vi "Measurement UI.vi"() -> ()   [LabVIEW 2021, in "Efficiency And Load Regulation with Pin Map UI.lvlib"]
uses:
  Efficiency And Load Regulation with Pin Map UI.lvlib
  <instrlib>/niScope/Controls/niScope vertical coupling.ctl
  <instrlib>/niDMM/nidmm.llb/niDMM Resolution in Digits.ctl
  subVIs/UI Controls.ctl
  common/UI/controls/UI Scope Parameters.ctl
  common/UI/controls/UI DMM Parameters.ctl
  d93153ab-98af-4bc3-81b9-2719e6b72da3.vi
  common/PMIC Common.lvlib
panel:
  in  "MeasGraphs":T1(tab)
  out "EfficiencyGraph 2":T2(graph)
  out "EfficiencyGraph":T2(graph)
  out "LoadRegulationGraph(V/A)":T2(graph)
  out "LoadRegulationGraph(%)":T2(graph)
  in  "dmm function array":u32[](array[ring]) items=["DC Volts", "AC Volts", "DC Current", "AC Current", "2-wire Resistance", "4-wire Resistance", "Diode", "Frequency", "Period", "AC Volts DC Coupled", "Capacitance", "Inductance", "Temperature"]
  in  "dmm range array":dbl[](array[numeric])
  in  "dmm resolution in digits array":T3[](array[typedef]) items=["3 1/2"=3.5, "4 1/2"=4.5, "5 1/2"=5.5, "6 1/2"=6.5, "7 1/2"=7.5]
  in  "dmm pin names":string[](array[string])
  in  "Source voltage array size":i32[](array[numeric])
  in  "Source voltage concatenated array":dbl[](array[numeric]) caption="VOLTAGE ARRAY"
  out "waveform pins":string[](array[string])
  in  "enforce realtime":bool[](array[boolean])
  in  "reference position":dbl[](array[numeric]) caption="MIN SAMPLE RATE"
  in  "channel enabled":bool[](array[boolean])
  out "waveform length array":i32[](array[numeric])
  out "waveform dt array":dbl[](array[numeric])
  out "Maximum load regulation":dbl[](array[numeric])
  out "Minimum load regulation":dbl[](array[numeric])
  out "Maximum load voltage":dbl[](array[numeric])
  out "Minimum load voltage":dbl[](array[numeric])
  out "Maximum efficiency":dbl[](array[numeric])
  out "Minimum efficiency":dbl[](array[numeric])
  out "Source sweep points":i32
  out "Load voltage deviation":dbl[](array[numeric])
  out "Load voltages":dbl[](array[numeric])
  out "Voltage values":dbl[](array[numeric])
  out "Load sweep points":i32
  out "Efficiency":dbl[](array[numeric])
  out "Load currents":dbl[](array[numeric])
  out "concatenated waveform Y":dbl[](array[numeric])
  out "waveform t0 array":dbl[](array[numeric])
  out "waveform sites":i32[](array[numeric])
  in  "vertical range":dbl[](array[numeric]) caption="VERTICAL RANGE"
  in  "vertical offset":dbl[](array[numeric]) caption="VERTICAL OFFSET"
  in  "probe attenuation":dbl[](array[numeric]) caption="PROBE ATTENUATION"
  in  "vertical coupling":T4[](array[typedef]) caption="VERTICAL COUPLING" items=["AC", "DC", "Ground"]
  in  "input impedance":u32[](array[ring]) caption="INPUT IMPEDANCE" items=["1 mega ohm"=0, "50 ohms"=2]
  in  "max input frequency":dbl[](array[numeric]) caption="MAX INPUT FREQUENCY"
  in  "min sample rate":dbl[](array[numeric]) caption="MIN SAMPLE RATE"
  in  "min record length":i32[](array[numeric]) caption="MIN RECORD LENGTH"
  in  "Pin Names for Scope":string[](array[string]) caption="PIN NAMES"
  out "MeasTable":string[][](table)
  in  "Source pin name index for efficiency":i32 caption="PIN INDEX USED IN EFFICIENCY CALCULATION"
  in  "Source stop voltage array":dbl[](array[numeric])=[20.0] caption="STOP VOLTAGE" format="%#_6pV"
  in  "Source start voltage array":dbl[](array[numeric])=[6.0] caption="START VOLTAGE" format="%#_6pV"
  in  "Source maximum power array":dbl[](array[numeric])=[300.0] caption="SOURCE MAXIMUM POWER" format="%#_6pW"
  in  "Source current limit array":dbl[](array[numeric])=[25.0] caption="SOURCE CURRENT LIMIT" format="%#_6pA"
  in  "Source sense array":i32[](array[ring])=[1009] caption="SOURCE SENSE" items=["Local"=1008, "Remote"=1009]
  in  "Source pin name array":string[](array[string]) caption="SOURCE PIN NAMES"
  in  "Open DMM Dialog":bool
  in  "DMM configuration":string="DMM configuration"
  in  "Open Scope Dialog":bool
  in  "Load pin name":string caption="LOAD PIN NAME"
  in  "Use Load current array":bool caption="USE ARRAY?"
  in  "Load current array":dbl[](array[numeric]) caption="CURRENT ARRAY"
  in  "Source voltage array":dbl[][](array[numeric]) caption="VOLTAGE ARRAY"
  in  "Use Source voltage array":bool caption="USE ARRAY?"
  in  "Scope configuration":string="Scope configuration"
  in  "Load sense":i32(ring)=1009 caption="SENSE" items=["Local"=1008, "Remote"=1009]
  out "Status":string
  in  "Load sweep type":string(combo)="Logarithmic" caption="SWEEP TYPE"
  in  "DUT setup time":dbl=1.0 caption="DUT SETUP TIME" format="%#_6ps"
  in  "Source voltage sweep points":i32=4 caption="NO. OF POINTS"
  in  "Aperture time":dbl=0.005 caption="APERTURE TIME" format="%#_6ps"
  in  "Source delay":dbl=0.005 caption="SOURCE DELAY" format="%#_6ps"
  in  "Load current sweep points/points per decade":i32=10 caption="PTS/PTS PER DECADE"
  in  "Load stop current":dbl=24.0 caption="STOP CURRENT" format="%#_6pA"
  in  "Load start current":dbl=0.1 caption="START CURRENT" format="%#_6pA"
  in  "Load voltage limit range":dbl=6.0 caption="VOLTAGE LIMIT RANGE" format="%#_6pV"
  in  "Load configuration":string="Load configuration"
  in  "Source configuration":string="Source configuration"
  in  "Measurement settings":string="Measurement settings"
  in  "Nominal output voltage":dbl=3.3 caption="NOMINAL OUTPUT VOLTAGE" format="%#_6pV"
  in  "Mode of operation":T5(ring)=enum."Perform measurement" caption="MODE OF OPERATION"
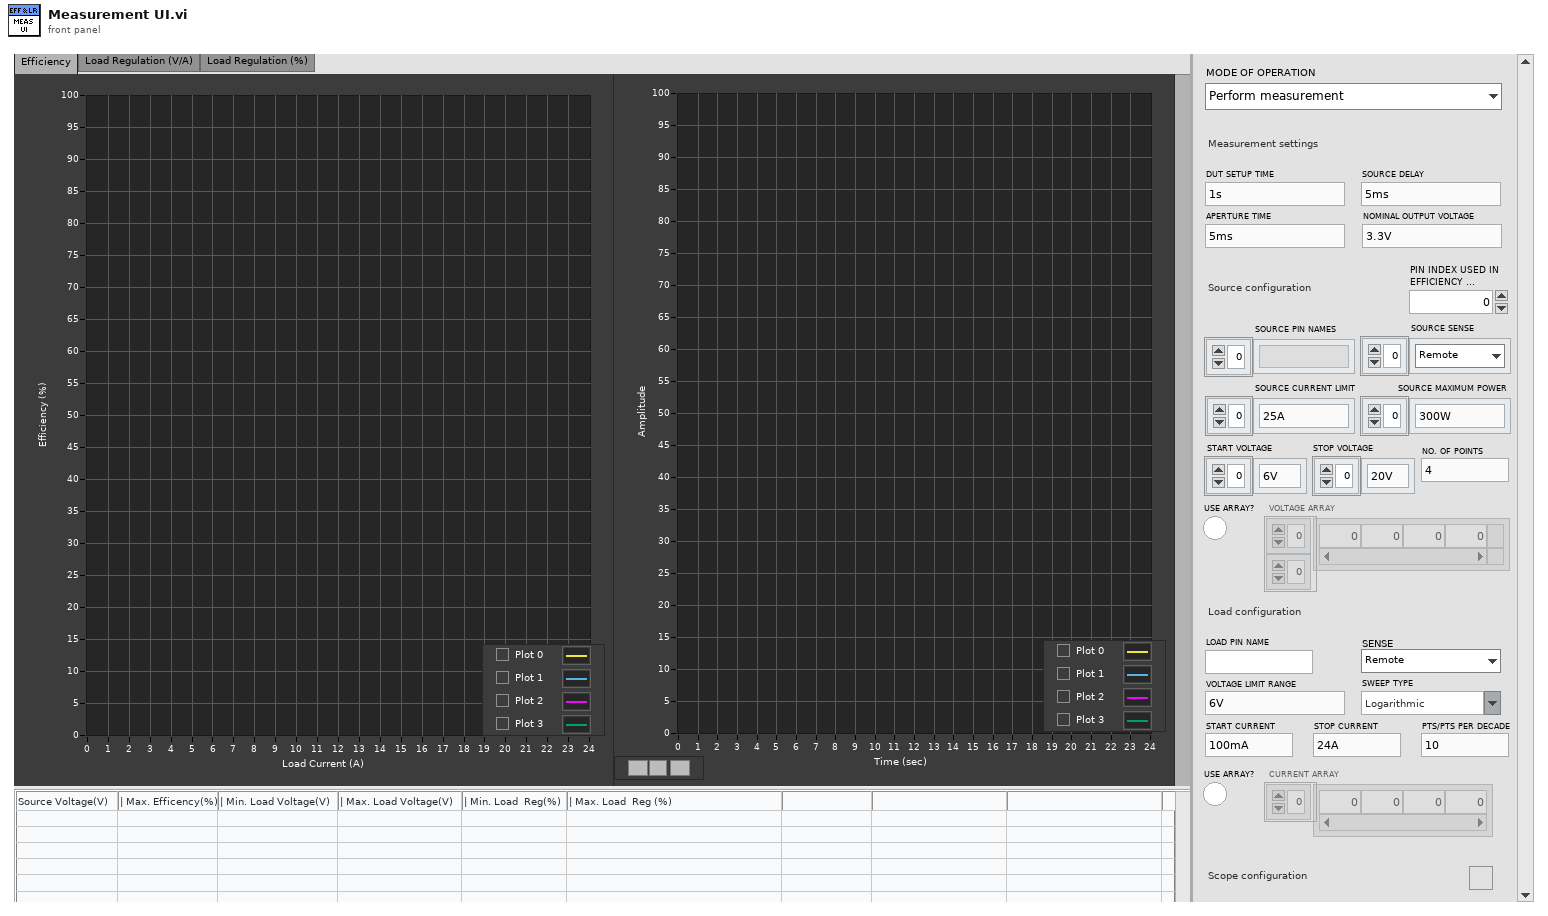
[diagram p1: front panel]
types:
  T1 = enum32{"Efficiency", "Load Regulation (V/A)", "Load Regulation (%)", "Hidden Controls"}
  T2 = cluster{"Load currents":dbl[], "Efficiency":dbl[]}[]
  T3 = typedef "niDMM Resolution in Digits.ctl" = dbl
  T4 = typedef "niScope vertical coupling.ctl" = i32
  T5 = enum32{"Power on the DUT", "Perform measurement", "Power off the DUT"}
  T6 = typedef "PMIC Common.lvlib/UI Scope Parameters.ctl" = cluster{"Pin name":string, "Vertical range":dbl, "Vertical offset":dbl, "Probe attenuation":dbl, "Vertical coupling":i32, "Channel enabled":bool, "Input impedance":u32, "Max input frequency":dbl, "Min sample rate":dbl, "Reference position":dbl, "Min record length":i32, "Enforce realtime":bool}
  T7 = typedef "PMIC Common.lvlib/UI DMM Parameters.ctl" = cluster{"Pin name":string, "Function":u32, "Resolution in Digits":dbl, "Range":dbl}
  T8 = enum8{"Enabled", "Disabled", "Disabled and Grayed Out"}
  T9 = typedef "Efficiency And Load Regulation with Pin Map UI.lvlib/UI Controls.ctl" = enum16{"", "EfficiencyGraph", "LoadRegulationGraph(V/A)", "LoadRegulationGraph(%)", "ScopeGraph", "DUT setup time", "Source delay", "Aperture time", "Nominal output voltage", "Source pin name", "Source current limit", "Source maximum power", "Source start voltage", "Source stop voltage", "Source voltage sweep points", "Load pin name", "Load voltage limit range", "Load sweep type", "Load start current", "Load stop current", "Load current sweep points/points per decade", "Use Load current array", "Load current array", "Use Source voltage array", "Source voltage array", "Pin Names for Scope", "vertical range", "vertical offset", "probe attenuation", "vertical coupling", "channel enabled", "input impedance", "max input frequency", "min sample rate", "reference position", "min record length", "enforce realtime", "Measurement settings", "Source configuration", "Load configuration", "Source sense", "Load sense", "Scope configuration", "Open Scope Dialog", "DMM configuration", "Open DMM Dialog", "Source pin name index for efficiency"}
  T10 = cluster{"Load currents":dbl[], "Efficiency":dbl[]}
  T11 = cluster{"Load currents":dbl[], "Load voltages":dbl[]}
  T12 = cluster{"Load currents":dbl[], "Load voltage deviation":dbl[]}
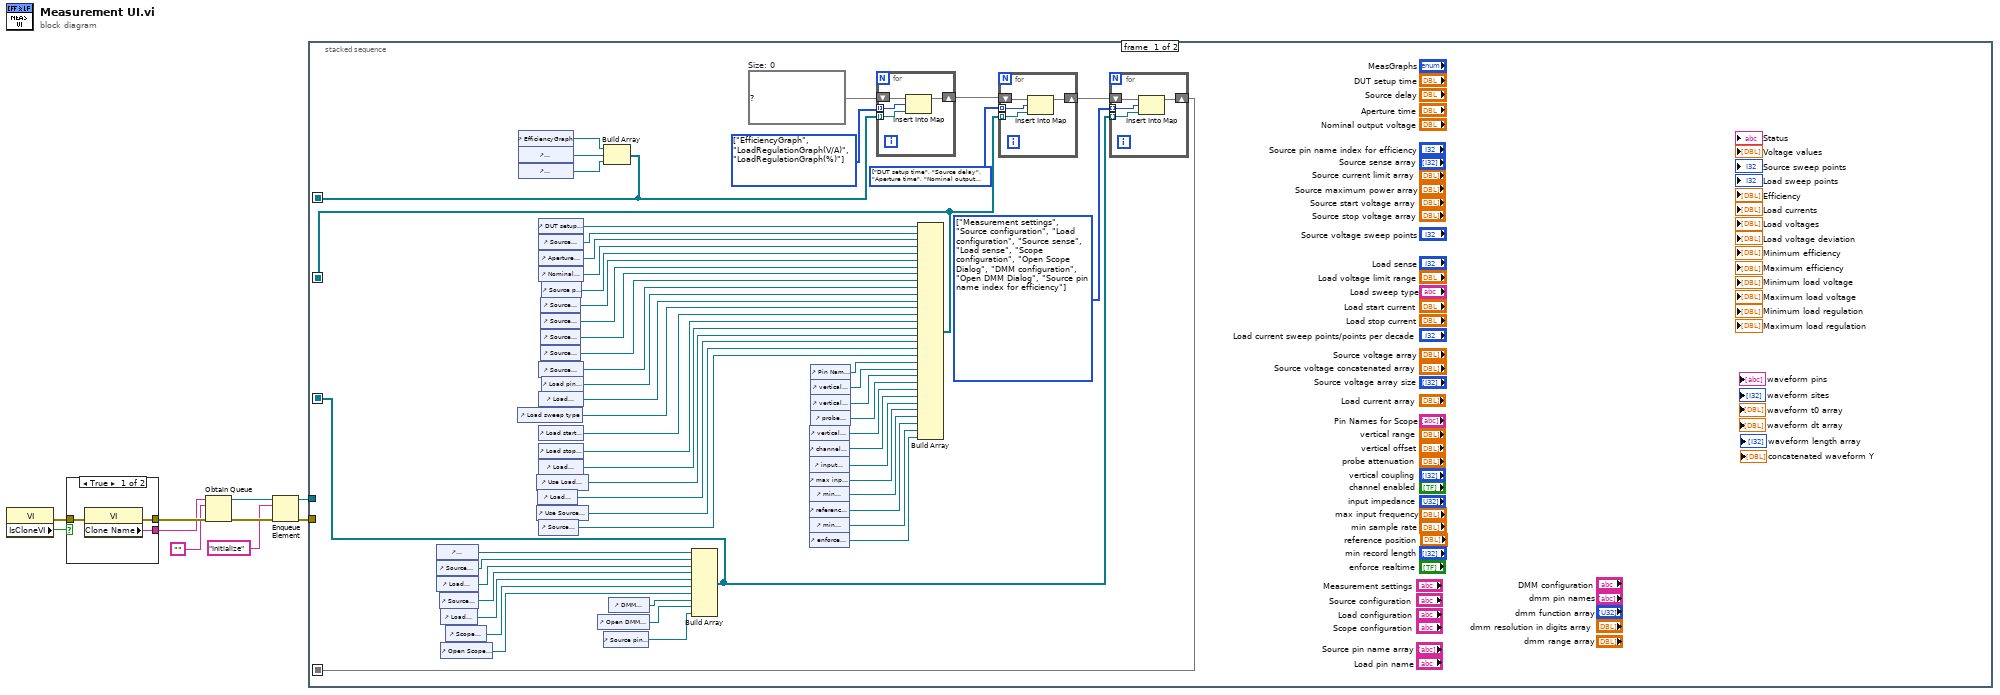
[diagram p0: block diagram]
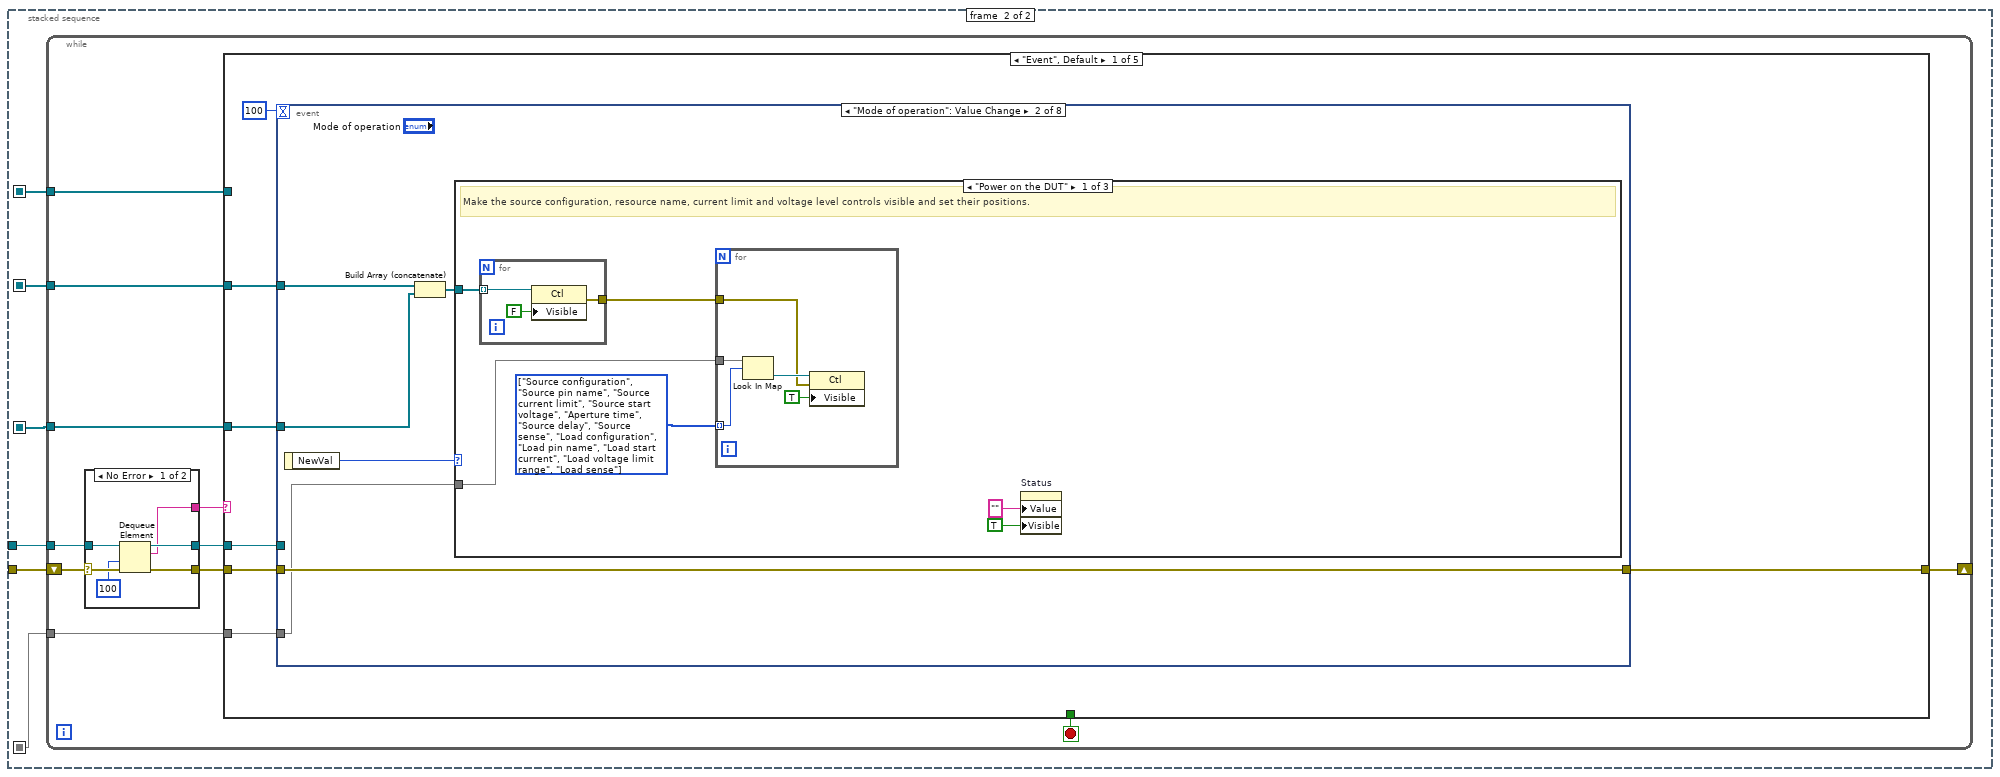
[diagram p2: hidden frame]
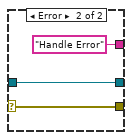
[diagram p3: hidden frame]
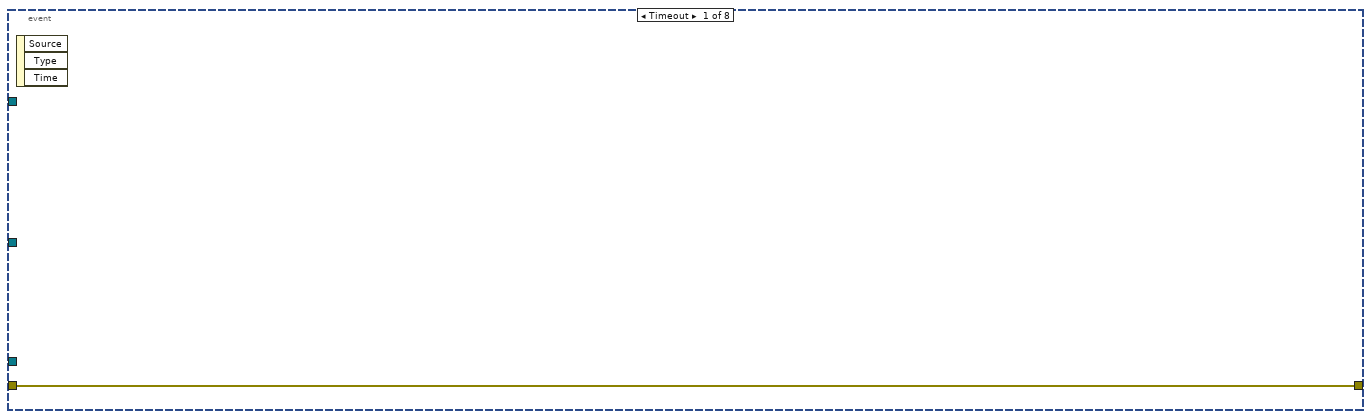
[diagram p4: hidden frame]
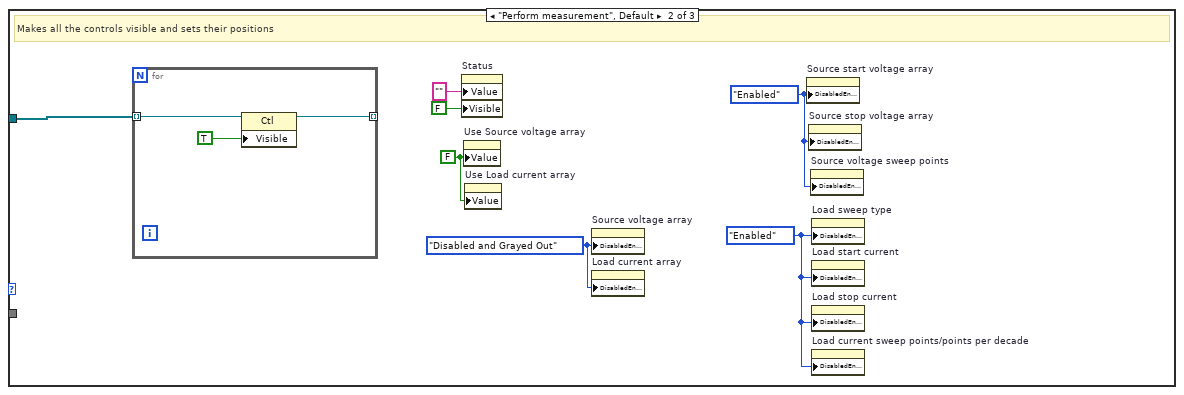
[diagram p5: hidden frame]
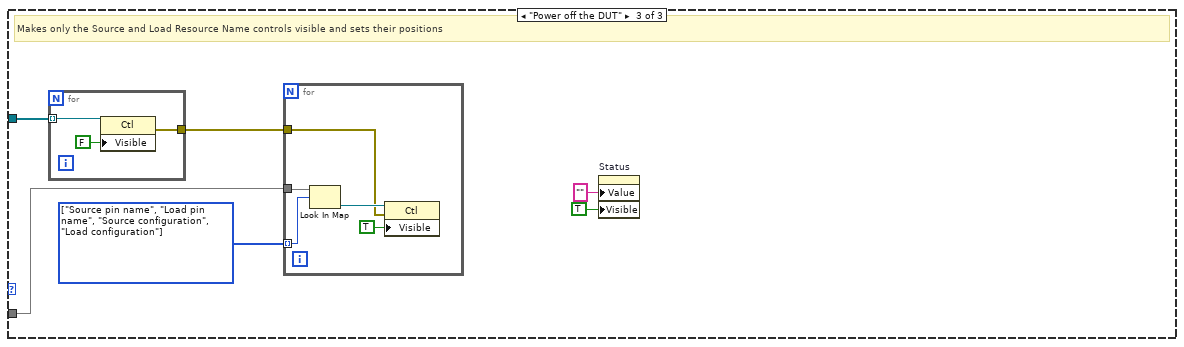
[diagram p6: hidden frame]
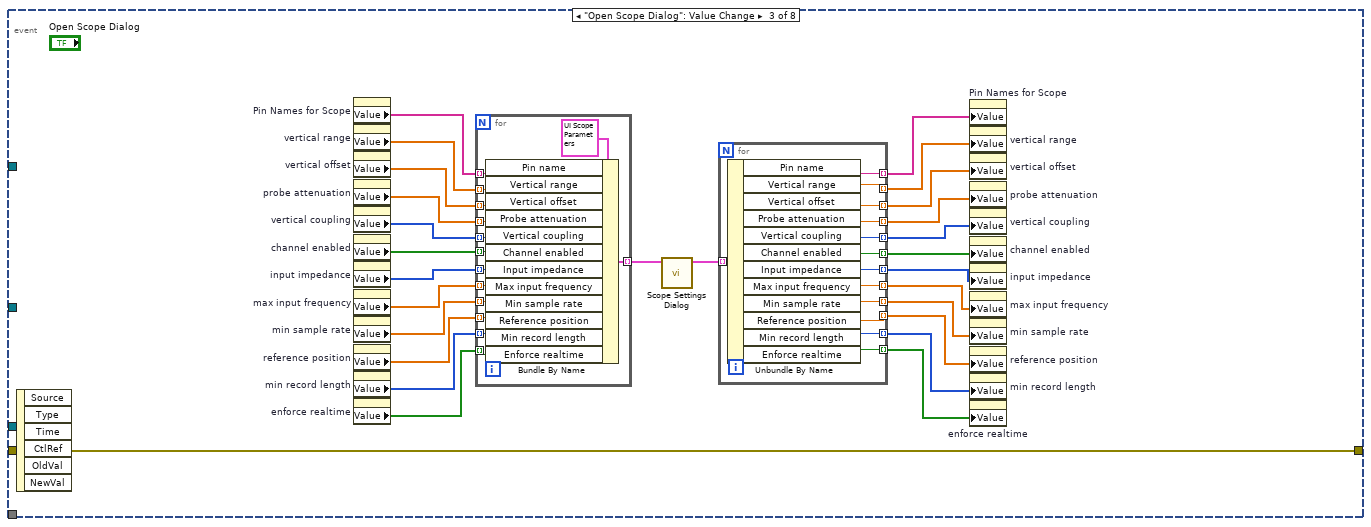
[diagram p7: hidden frame]
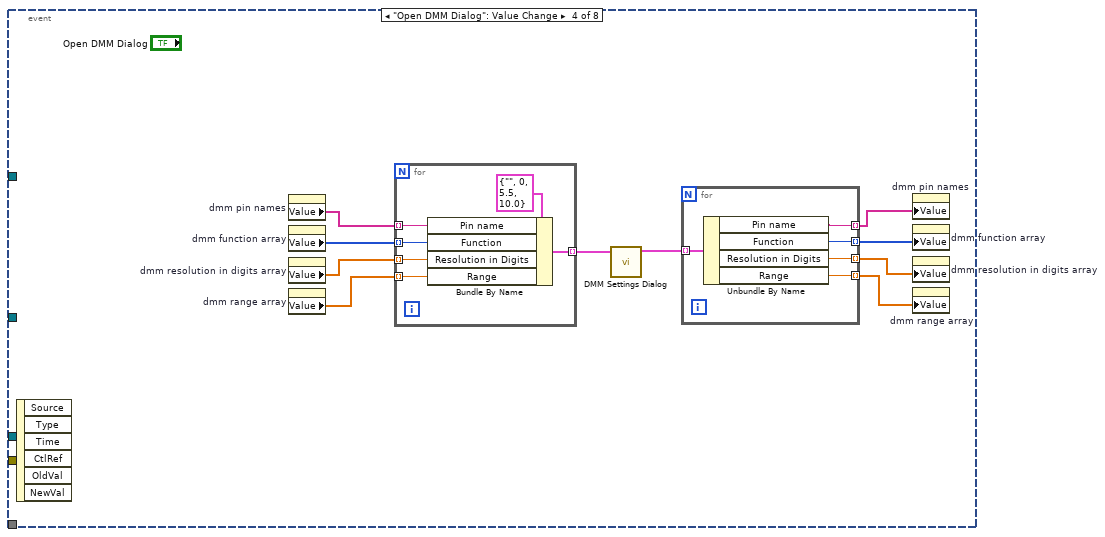
[diagram p8: hidden frame]
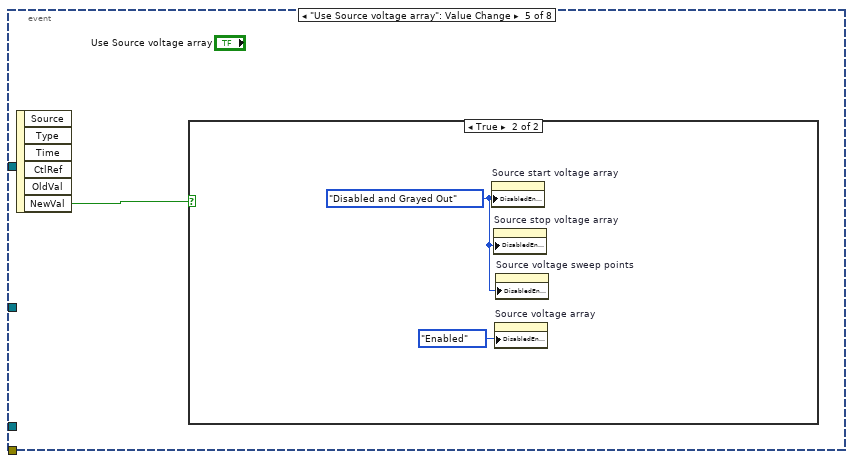
[diagram p9: hidden frame]
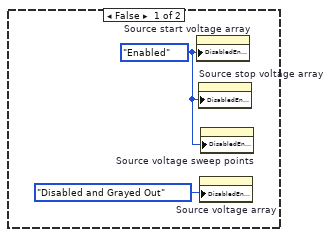
[diagram p10: hidden frame]
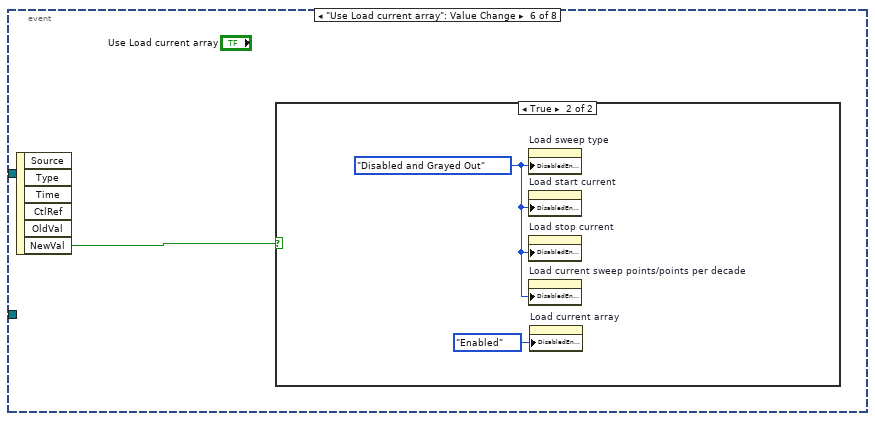
[diagram p11: hidden frame]
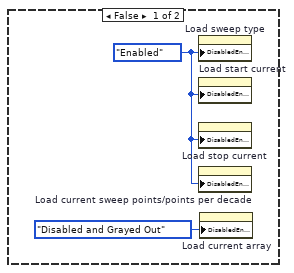
[diagram p12: hidden frame]
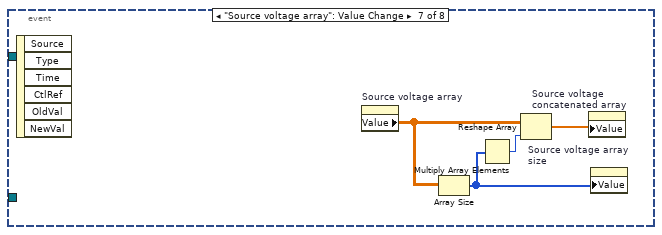
[diagram p13: hidden frame]
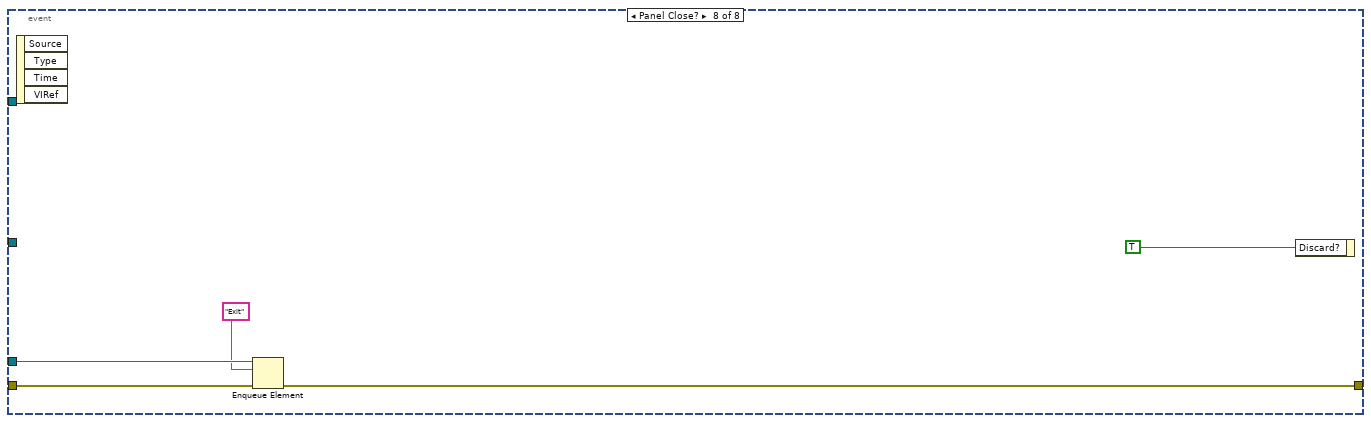
[diagram p14: hidden frame]
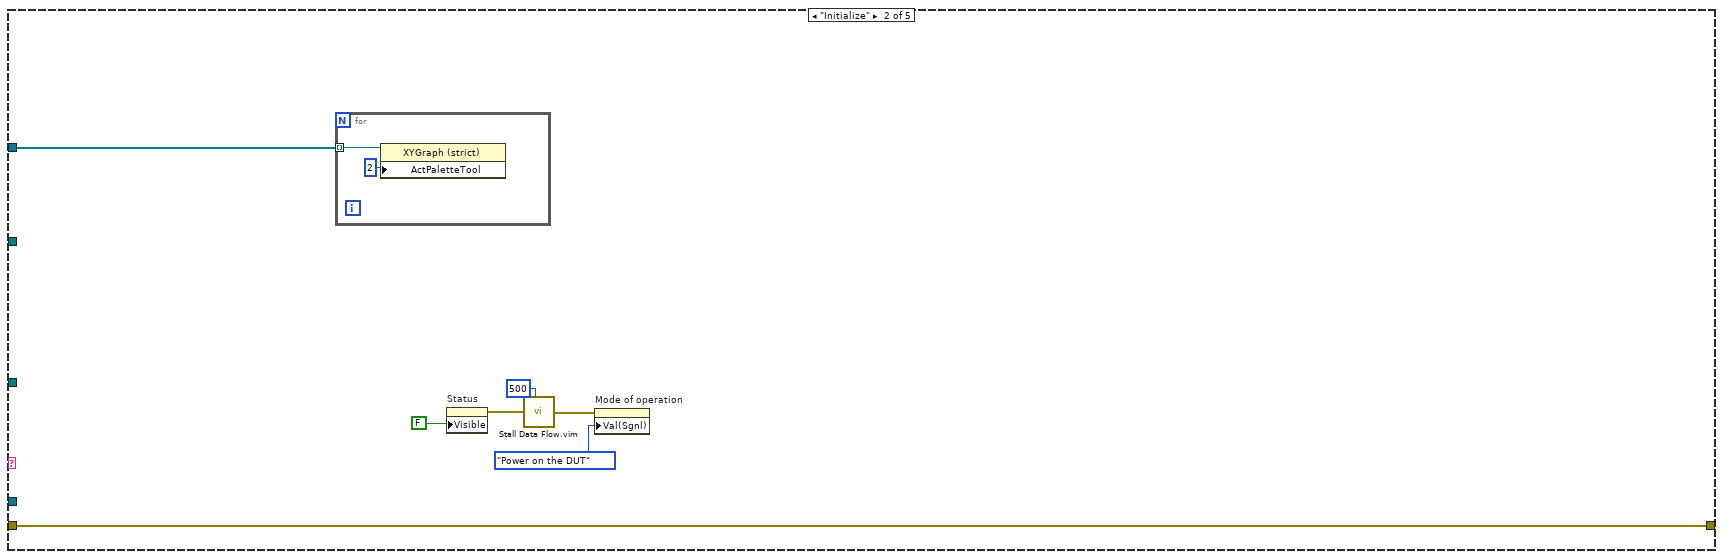
[diagram p15: hidden frame]
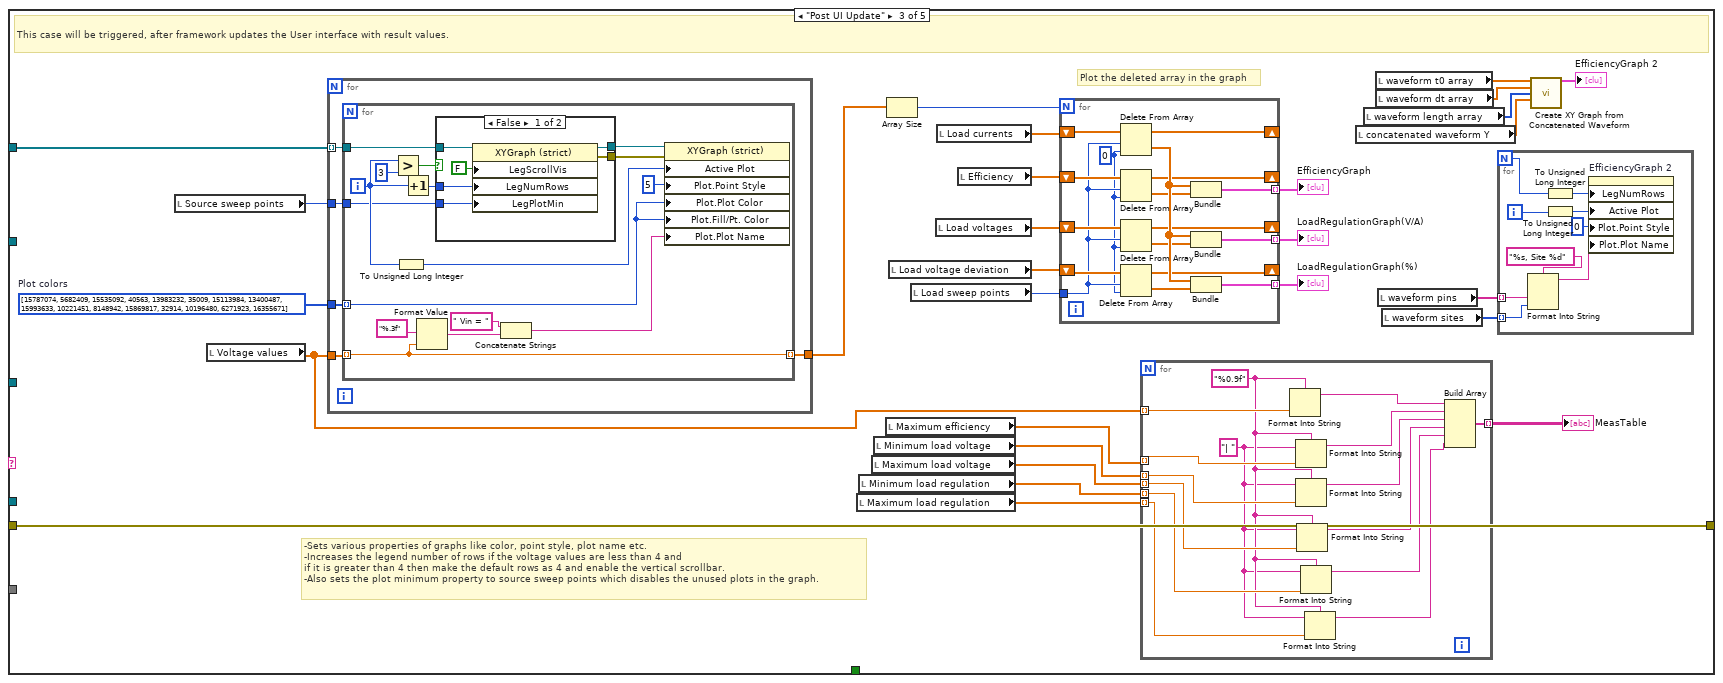
[diagram p16: hidden frame]
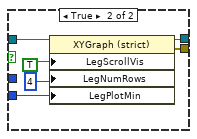
[diagram p17: hidden frame]
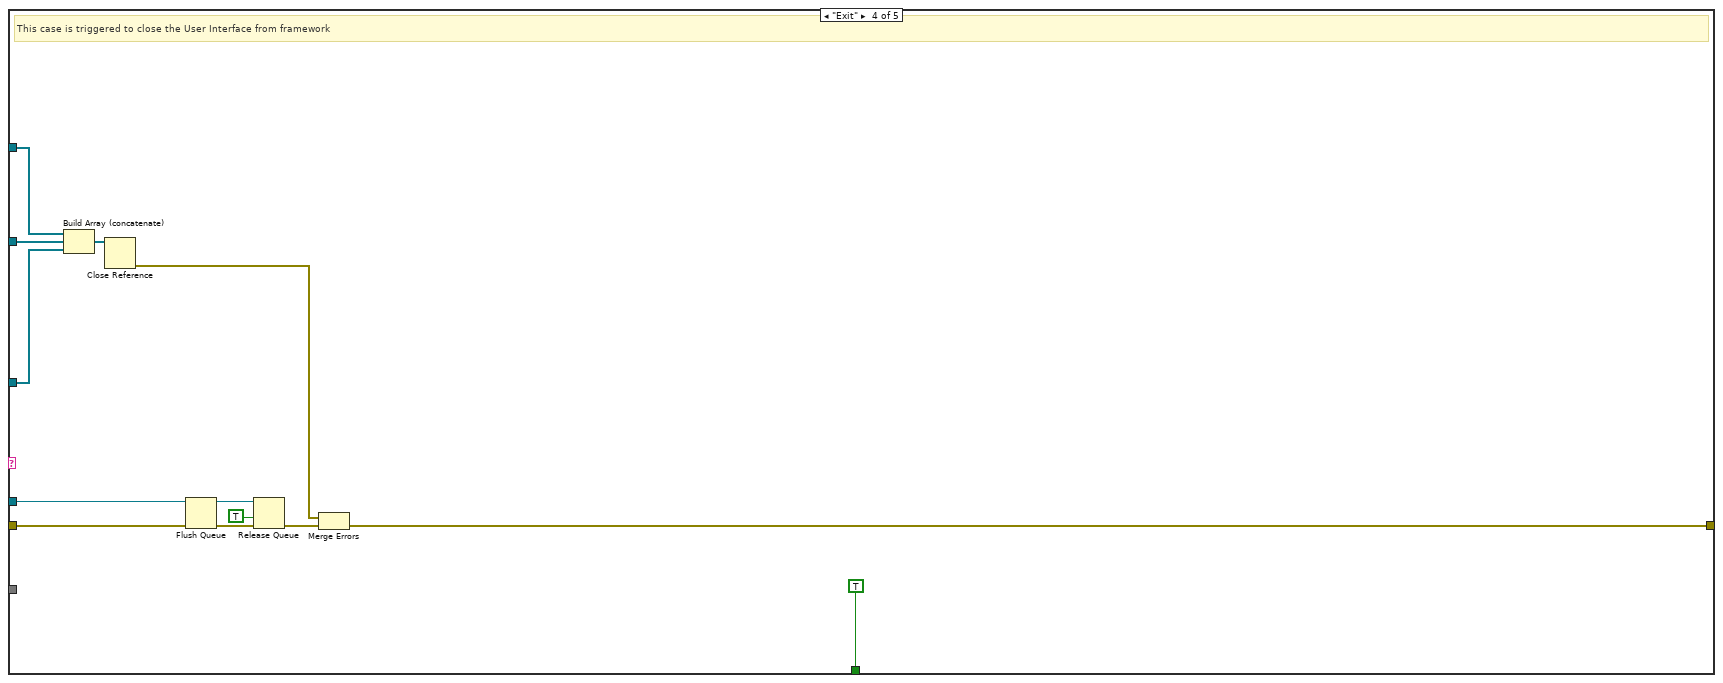
[diagram p18: hidden frame]
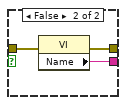
[diagram p20: hidden frame]
diagram:
  n1 = property class="VI"() -> (error out=w1:errorcluster, "IsCloneVI"=w2:bool)  [unwired: 2 in, 1 out]
  n2 = case shown="True" w2 {
    tunnel: [w13 w16] -> w10
    tunnel: [w12 w15] -> w9
    tunnel: w1 -> [w11 w14]
    frame True {
      n3 = property class="VI"(error in=w11) -> (error out=w13:errorcluster, "Clone Name"=w12:string)  [unwired: 1 in, 1 out]
    }
    frame False {
      n4 = property class="VI"(error in=w14) -> (error out=w16:errorcluster, "Name"=w15:string)  [unwired: 1 in, 1 out]
    }
  }
  n5 = Obtain Queue(name (unnamed)=w9, element data type="", error in (no error)=w10) -> (queue out=w6:refnum<queue>, error out=w8:errorcluster)  [unwired: 2 in, 1 out]
  n6 = Enqueue Element(queue=w6, element="Initialize", error in (no error)=w8) -> (queue out=w5:refnum<queue>, error out=w7:errorcluster)  [unwired: 1 in, 1 out]
  n7 = stacked-sequence {
    seq-local: [w43 _] -> [_ w87]
    seq-local: [w31 _] -> [_ w86]
    seq-local: [w30 _] -> [_ w85]
    seq-local: [w29 _] -> [_ w84]
    tunnel: w7 -> [_ w89]
    tunnel: w5 -> [_ w88]
    frame #0 {
      w23 = map{T9, refnum<vi>} {}  # Size: 0
      w24 = T9[] [enum."Measurement settings", enum."Source configuration", enum."Load configuration", enum."Source sense", enum."Load sense", enum."Scope configuration", enum."Open Scope Dialog", enum."DMM configuration", enum."Open DMM Dialog", enum."Source pin name index for efficiency"] items=["", "EfficiencyGraph", "LoadRegulationGraph(V/A)", "LoadRegulationGraph(%)", "ScopeGraph", "DUT setup time", "Source delay", "Aperture time", "Nominal output voltage", "Source pin name", "Source current limit", "Source maximum power", "Source start voltage", "Source stop voltage", "Source voltage sweep points", "Load pin name", "Load voltage limit range", "Load sweep type", "Load start current", "Load stop current", "Load current sweep points/points per decade", "Use Load current array", "Load current array", "Use Source voltage array", "Source voltage array", "Pin Names for Scope", "vertical range", "vertical offset", "probe attenuation", "vertical coupling", "channel enabled", "input impedance", "max input frequency", "min sample rate", "reference position", "min record length", "enforce realtime", "Measurement settings", "Source configuration", "Load configuration", "Source sense", "Load sense", "Scope configuration", "Open Scope Dialog", "DMM configuration", "Open DMM Dialog", "Source pin name index for efficiency"]
      w26 = T9[] [enum."DUT setup time", enum."Source delay", enum."Aperture time", enum."Nominal output voltage", enum."Source pin name", enum."Source current limit", enum."Source maximum power", enum."Source start voltage", enum."Source stop voltage", enum."Source voltage sweep points", enum."Load pin name", enum."Load voltage limit range", enum."Load sweep type", enum."Load start current", enum."Load stop current", enum."Load current sweep points/points per decade", enum."Use Load current array", enum."Load current array", enum."Use Source voltage array", enum."Source voltage array", enum."Pin Names for Scope", enum."vertical range", enum."vertical offset", enum."probe attenuation", enum."vertical coupling", enum."channel enabled", enum."input impedance", enum."max input frequency", enum."min sample rate", enum."reference position", enum."min record length", enum."enforce realtime"] items=["", "EfficiencyGraph", "LoadRegulationGraph(V/A)", "LoadRegulationGraph(%)", "ScopeGraph", "DUT setup time", "Source delay", "Aperture time", "Nominal output voltage", "Source pin name", "Source current limit", "Source maximum power", "Source start voltage", "Source stop voltage", "Source voltage sweep points", "Load pin name", "Load voltage limit range", "Load sweep type", "Load start current", "Load stop current", "Load current sweep points/points per decade", "Use Load current array", "Load current array", "Use Source voltage array", "Source voltage array", "Pin Names for Scope", "vertical range", "vertical offset", "probe attenuation", "vertical coupling", "channel enabled", "input impedance", "max input frequency", "min sample rate", "reference position", "min record length", "enforce realtime", "Measurement settings", "Source configuration", "Load configuration", "Source sense", "Load sense", "Scope configuration", "Open Scope Dialog", "DMM configuration", "Open DMM Dialog", "Source pin name index for efficiency"]
      w28 = T9[] [enum."EfficiencyGraph", enum."LoadRegulationGraph(V/A)", enum."LoadRegulationGraph(%)"] items=["", "EfficiencyGraph", "LoadRegulationGraph(V/A)", "LoadRegulationGraph(%)", "ScopeGraph", "DUT setup time", "Source delay", "Aperture time", "Nominal output voltage", "Source pin name", "Source current limit", "Source maximum power", "Source start voltage", "Source stop voltage", "Source voltage sweep points", "Load pin name", "Load voltage limit range", "Load sweep type", "Load start current", "Load stop current", "Load current sweep points/points per decade", "Use Load current array", "Load current array", "Use Source voltage array", "Source voltage array", "Pin Names for Scope", "vertical range", "vertical offset", "probe attenuation", "vertical coupling", "channel enabled", "input impedance", "max input frequency", "min sample rate", "reference position", "min record length", "enforce realtime", "Measurement settings", "Source configuration", "Load configuration", "Source sense", "Load sense", "Scope configuration", "Open Scope Dialog", "DMM configuration", "Open DMM Dialog", "Source pin name index for efficiency"]
      n8 = control-ref of="Measurement settings"() -> (w57:refnum<vi>)
      n9 = control-ref of="Source configuration"() -> (w55:refnum<vi>)
      n10 = control-ref of="Load configuration"() -> (w56:refnum<vi>)
      n11 = control-ref of="Source sense array"() -> (w51:refnum<vi>)
      n12 = control-ref of="Load sense"() -> (w50:refnum<vi>)
      n13 = control-ref of="Open Scope Dialog"() -> (w20:refnum<vi>)
      n14 = control-ref of="Scope configuration"() -> (w48:refnum<vi>)
      n15 = control-ref of="Load sweep type"() -> (w62:refnum<vi>)
      n16 = control-ref of="EfficiencyGraph"() -> (w54:refnum<vi>)
      n17 = control-ref of="LoadRegulationGraph(V/A)"() -> (w53:refnum<vi>)
      n18 = control-ref of="LoadRegulationGraph(%)"() -> (w52:refnum<vi>)
      n19 = control-ref of="Use Load current array"() -> (w47:refnum<vi>)
      n20 = control-ref of="Use Source voltage array"() -> (w45:refnum<vi>)
      n21 = control-ref of="Load current array"() -> (w46:refnum<vi>)
      n22 = control-ref of="DUT setup time"() -> (w71:refnum<vi>)
      n23 = control-ref of="Source delay"() -> (w70:refnum<vi>)
      n24 = control-ref of="Aperture time"() -> (w69:refnum<vi>)
      n25 = control-ref of="Nominal output voltage"() -> (w58:refnum<vi>)
      n26 = control-ref of="Source voltage sweep points"() -> (w64:refnum<vi>)
      n27 = control-ref of="Load voltage limit range"() -> (w63:refnum<vi>)
      n28 = control-ref of="Load start current"() -> (w61:refnum<vi>)
      n29 = control-ref of="Load stop current"() -> (w60:refnum<vi>)
      n30 = control-ref of="Load current sweep points/points per decade"() -> (w59:refnum<vi>)
      n31 = control-ref of="Source voltage array"() -> (w44:refnum<vi>)
      n32 = control-ref of="Source current limit array"() -> (w68:refnum<vi>)
      n33 = control-ref of="Source maximum power array"() -> (w67:refnum<vi>)
      n34 = control-ref of="Source start voltage array"() -> (w66:refnum<vi>)
      n35 = control-ref of="Source stop voltage array"() -> (w65:refnum<vi>)
      n36 = control-ref of="Source pin name array"() -> (w22:refnum<vi>)
      n37 = control-ref of="Load pin name"() -> (w21:refnum<vi>)
      n38 = control-ref of="Open DMM Dialog"() -> (w18:refnum<vi>)
      n39 = Build Array(w54, w53, w52) -> (w43:refnum<vi>[])
      n40 = control-ref of="Source pin name index for efficiency"() -> (w17:refnum<vi>)
      n41 = control-ref of="DMM configuration"() -> (w19:refnum<vi>)
      n42 = Build Array(w57, w55, w56, w51, w50, w48, w20, w19, w18, w17) -> (w30:refnum<vi>[])
      n43 = control-ref of="vertical coupling"() -> (w39:refnum<vi>)
      n44 = control-ref of="channel enabled"() -> (w38:refnum<vi>)
      n45 = control-ref of="input impedance"() -> (w37:refnum<vi>)
      n46 = control-ref of="max input frequency"() -> (w36:refnum<vi>)
      n47 = control-ref of="min sample rate"() -> (w35:refnum<vi>)
      n48 = control-ref of="reference position"() -> (w34:refnum<vi>)
      n49 = control-ref of="min record length"() -> (w33:refnum<vi>)
      n50 = control-ref of="enforce realtime"() -> (w32:refnum<vi>)
      n51 = control-ref of="Pin Names for Scope"() -> (w49:refnum<vi>)
      n52 = control-ref of="vertical range"() -> (w42:refnum<vi>)
      n53 = control-ref of="vertical offset"() -> (w41:refnum<vi>)
      n54 = control-ref of="probe attenuation"() -> (w40:refnum<vi>)
      n55 = for {
        shift-right: [w82] -> w27
        shift-left: w23 -> [w83]
        tunnel: w28 -> [w81] mode=indexing
        tunnel: w43 -> [w80] mode=indexing
        n56 = Insert Into Map(map in=w83, key=w81, value=w80) -> (map out=w82:map{T9, refnum<vi>})  [unwired: 2 out]
      }
      n57 = Build Array(w71, w70, w69, w58, w22, w68, w67, w66, w65, w64, w21, w63, w62, w61, w60, w59, w47, w46, w45, w44, w49, w42, w41, w40, w39, w38, w37, w36, w35, w34, w33, w32) -> (w31:refnum<vi>[])
      n58 = for {
        shift-right: [w78] -> w25
        shift-left: w27 -> [w79]
        tunnel: w26 -> [w77] mode=indexing
        tunnel: w31 -> [w76] mode=indexing
        n59 = Insert Into Map(map in=w79, key=w77, value=w76) -> (map out=w78:map{T9, refnum<vi>})  [unwired: 2 out]
      }
      n60 = for {
        shift-right: [w74] -> w29
        shift-left: w25 -> [w75]
        tunnel: w24 -> [w73] mode=indexing
        tunnel: w30 -> [w72] mode=indexing
        n61 = Insert Into Map(map in=w75, key=w73, value=w72) -> (map out=w74:map{T9, refnum<vi>})  [unwired: 2 out]
      }
    }
    frame #1 {
      n62 = while {
        shift-right: [w95] -> _
        shift-left: w89 -> [w100]
        tunnel: w88 -> [w98]
        tunnel: w86 -> [w93]
        tunnel: w85 -> [w92]
        tunnel: w87 -> [w91]
        tunnel: w84 -> [w90]
        stop <- w94 stop-if-true
        n63 = case shown="No Error" w100 {
          selector: w100 -> [w106 w109]
          tunnel: [w105 w109] -> w99
          tunnel: w98 -> [w104 w108]
          tunnel: [w103 w108] -> w97
          tunnel: [w102 "Handle Error"] -> w96
          frame No Error {
            n64 = Dequeue Element(queue=w104, timeout in ms (-1)=100, error in (no error)=w106) -> (queue out=w103:refnum<queue>, element=w102:string, error out=w105:errorcluster)  [unwired: 1 out]
          }
          frame Error {
          }
        }
        n65 = case shown="\"Event\", Default" w96 {
          tunnel: w99 -> [w115 w262 w292 w379 w380]
          tunnel: w97 -> [w113 _ _ w377 _]
          tunnel: [w116 w262 w292 w371 w380] -> w95
          tunnel: [_ _ _ TRUE _] -> w94
          tunnel: w93 -> [w112 _ _ w369 _]
          tunnel: w92 -> [w111 _ _ w368 _]
          tunnel: w91 -> [_ w261 w282 w370 _]
          tunnel: w90 -> [w110 _ _ _ _]
          frame "Event", Default {
            n66 = event shown="[1] \"Mode of operation\": Value Change" {
              selector: _ -> [_ _ _ _ _ _ _ _]
              dyn-events: _ -> [_ _ _ _ _ _ _ _]
              timeout: 100 -> [_ _ _ _ _ _ _ _]
              tunnel: [w117 w120 w162 _ _ _ _ w253] -> w116
              tunnel: w115 -> [w117 w120 w162 _ _ _ _ w254]
              tunnel: w113 -> [_ _ _ _ _ _ _ w252]
              tunnel: w112 -> [_ w121 _ _ _ _ _ _]
              tunnel: w111 -> [_ w122 _ _ _ _ _ _]
              tunnel: w110 -> [_ w119 _ _ _ _ _ _]
              event Timeout {
                n67 = event-data() -> ()  [unwired: 1 in, 3 out]
              }
              event "Mode of operation": Value Change {
                n68 = event-data() -> ("NewVal"=w123:T5)  [unwired: 1 in]
                n69 = Build Array (concatenate)(w121, w122) -> (w118:refnum<vi>[])
                n70 = case shown="\"Power on the DUT\"" w123 {
                  tunnel: w118 -> [w129 w144 w153]
                  tunnel: w119 -> [w126 _ w150]
                  frame "Power on the DUT" {
                    w125 = T9[] [enum."Source configuration", enum."Source pin name", enum."Source current limit", enum."Source start voltage", enum."Aperture time", enum."Source delay", enum."Source sense", enum."Load configuration", enum."Load pin name", enum."Load start current", enum."Load voltage limit range", enum."Load sense"] items=["", "EfficiencyGraph", "LoadRegulationGraph(V/A)", "LoadRegulationGraph(%)", "ScopeGraph", "DUT setup time", "Source delay", "Aperture time", "Nominal output voltage", "Source pin name", "Source current limit", "Source maximum power", "Source start voltage", "Source stop voltage", "Source voltage sweep points", "Load pin name", "Load voltage limit range", "Load sweep type", "Load start current", "Load stop current", "Load current sweep points/points per decade", "Use Load current array", "Load current array", "Use Source voltage array", "Source voltage array", "Pin Names for Scope", "vertical range", "vertical offset", "probe attenuation", "vertical coupling", "channel enabled", "input impedance", "max input frequency", "min sample rate", "reference position", "min record length", "enforce realtime", "Measurement settings", "Source configuration", "Load configuration", "Source sense", "Load sense", "Scope configuration", "Open Scope Dialog", "DMM configuration", "Open DMM Dialog", "Source pin name index for efficiency"]
                    # "Make the source configuration, resource name, current limit and voltage level controls visible and set their positions."
                    n71 = for {
                      tunnel: w129 -> [w132] mode=indexing
                      tunnel: [w130] -> w124
                      n72 = property class="Ctl"(reference=w132, "Visible"=FALSE) -> (error out=w130:errorcluster)  [unwired: 1 in, 1 out]
                    }
                    n73 = for {
                      tunnel: w126 -> [w135]
                      tunnel: w125 -> [w134] mode=indexing
                      tunnel: w124 -> [w133]
                      n74 = Look In Map(map=w135, key=w134) -> (value=w136:refnum<vi>)  [unwired: 1 in, 1 out]
                      n75 = property class="Ctl"(reference=w136, error in=w133, "Visible"=TRUE) -> ()  [unwired: 2 out]
                    }
                    n76 = property on="Status" class="Str"("Value"="" ("Status"), "Visible"=TRUE) -> ()  [unwired: 2 in, 2 out]
                  }
                  frame "Perform measurement", Default {
                    w138 = T8."Enabled" ("Disabled")
                    w139 = T8."Enabled" ("Disabled")
                    w140 = T8."Disabled and Grayed Out" ("Disabled")
                    w141 = FALSE ("Use Source voltage array")
                    # "Makes all the controls visible and sets their positions"
                    n77 = for {
                      tunnel: w144 -> [w145] mode=indexing
                      tunnel: [w146] -> _ mode=indexing
                      n78 = property class="Ctl"(reference=w145, "Visible"=TRUE) -> (reference out=w146:refnum<vi>)  [unwired: 1 in, 1 out]
                    }
                    n79 = property on="Status" class="Str"("Value"="" ("Status"), "Visible"=FALSE) -> ()  [unwired: 2 in, 2 out]
                    n80 = property on="Use Source voltage array" class="Bool (strict)"("Value"=w141) -> ()  [unwired: 2 in, 2 out]
                    n81 = property on="Use Load current array" class="Bool (strict)"("Value"=w141) -> ()  [unwired: 2 in, 2 out]
                    n82 = property on="Source voltage array" class="Arr (strict)"("DisabledEnum"=w140) -> ()  [unwired: 2 in, 2 out]
                    n83 = property on="Load current array" class="Arr (strict)"("DisabledEnum"=w140) -> ()  [unwired: 2 in, 2 out]
                    n84 = property on="Source start voltage array" class="Arr (strict)"("DisabledEnum"=w138) -> ()  [unwired: 2 in, 2 out]
                    n85 = property on="Source stop voltage array" class="Arr (strict)"("DisabledEnum"=w138) -> ()  [unwired: 2 in, 2 out]
                    n86 = property on="Source voltage sweep points" class="DigNum (strict)"("DisabledEnum"=w138) -> ()  [unwired: 2 in, 2 out]
                    n87 = property on="Load sweep type" class="CmbBox"("DisabledEnum"=w139) -> ()  [unwired: 2 in, 2 out]
                    n88 = property on="Load start current" class="DigNum (strict)"("DisabledEnum"=w139) -> ()  [unwired: 2 in, 2 out]
                    n89 = property on="Load stop current" class="DigNum (strict)"("DisabledEnum"=w139) -> ()  [unwired: 2 in, 2 out]
                    n90 = property on="Load current sweep points/points per decade" class="DigNum (strict)"("DisabledEnum"=w139) -> ()  [unwired: 2 in, 2 out]
                  }
                  frame "Power off the DUT" {
                    w149 = T9[] [enum."Source pin name", enum."Load pin name", enum."Source configuration", enum."Load configuration"] items=["", "EfficiencyGraph", "LoadRegulationGraph(V/A)", "LoadRegulationGraph(%)", "ScopeGraph", "DUT setup time", "Source delay", "Aperture time", "Nominal output voltage", "Source pin name", "Source current limit", "Source maximum power", "Source start voltage", "Source stop voltage", "Source voltage sweep points", "Load pin name", "Load voltage limit range", "Load sweep type", "Load start current", "Load stop current", "Load current sweep points/points per decade", "Use Load current array", "Load current array", "Use Source voltage array", "Source voltage array", "Pin Names for Scope", "vertical range", "vertical offset", "probe attenuation", "vertical coupling", "channel enabled", "input impedance", "max input frequency", "min sample rate", "reference position", "min record length", "enforce realtime", "Measurement settings", "Source configuration", "Load configuration", "Source sense", "Load sense", "Scope configuration", "Open Scope Dialog", "DMM configuration", "Open DMM Dialog", "Source pin name index for efficiency"]
                    # "Makes only the Source and Load Resource Name controls visible and sets their positions"
                    n91 = for {
                      tunnel: w153 -> [w155] mode=indexing
                      tunnel: [w154] -> w148
                      n92 = property class="Ctl"(reference=w155, "Visible"=FALSE) -> (error out=w154:errorcluster)  [unwired: 1 in, 1 out]
                    }
                    n93 = for {
                      tunnel: w150 -> [w160]
                      tunnel: w149 -> [w158] mode=indexing
                      tunnel: w148 -> [w157]
                      n94 = Look In Map(map=w160, key=w158) -> (value=w159:refnum<vi>)  [unwired: 1 in, 1 out]
                      n95 = property class="Ctl"(reference=w159, error in=w157, "Visible"=TRUE) -> ()  [unwired: 2 out]
                    }
                    n96 = property on="Status" class="Str"("Value"="" ("Status"), "Visible"=TRUE) -> ()  [unwired: 2 in, 2 out]
                  }
                }
              }
              event "Open Scope Dialog": Value Change {
                n97 = event-data() -> ()  [unwired: 1 in, 6 out]
                n98 = property on="Pin Names for Scope" class="Arr (strict)"() -> ("Value"=w175:string[])  [unwired: 2 in, 2 out]
                n99 = property on="vertical range" class="Arr (strict)"() -> ("Value"=w174:dbl[])  [unwired: 2 in, 2 out]
                n100 = property on="vertical offset" class="Arr (strict)"() -> ("Value"=w173:dbl[])  [unwired: 2 in, 2 out]
                n101 = property on="probe attenuation" class="Arr (strict)"() -> ("Value"=w172:dbl[])  [unwired: 2 in, 2 out]
                n102 = property on="vertical coupling" class="Arr (strict)"() -> ("Value"=w171:T4[])  [unwired: 2 in, 2 out]
                n103 = property on="channel enabled" class="Arr (strict)"() -> ("Value"=w170:bool[])  [unwired: 2 in, 2 out]
                n104 = property on="input impedance" class="Arr (strict)"() -> ("Value"=w169:u32[])  [unwired: 2 in, 2 out]
                n105 = property on="max input frequency" class="Arr (strict)"() -> ("Value"=w168:dbl[])  [unwired: 2 in, 2 out]
                n106 = property on="min sample rate" class="Arr (strict)"() -> ("Value"=w167:dbl[])  [unwired: 2 in, 2 out]
                n107 = property on="reference position" class="Arr (strict)"() -> ("Value"=w166:dbl[])  [unwired: 2 in, 2 out]
                n108 = property on="min record length" class="Arr (strict)"() -> ("Value"=w165:i32[])  [unwired: 2 in, 2 out]
                n109 = property on="enforce realtime" class="Arr (strict)"() -> ("Value"=w164:bool[])  [unwired: 2 in, 2 out]
                n110 = for {
                  tunnel: w175 -> [w202] mode=indexing
                  tunnel: w174 -> [w201] mode=indexing
                  tunnel: w173 -> [w200] mode=indexing
                  tunnel: w172 -> [w199] mode=indexing
                  tunnel: w171 -> [w198] mode=indexing
                  tunnel: w170 -> [w197] mode=indexing
                  tunnel: w169 -> [w196] mode=indexing
                  tunnel: w168 -> [w195] mode=indexing
                  tunnel: w167 -> [w194] mode=indexing
                  tunnel: w166 -> [w193] mode=indexing
                  tunnel: w165 -> [w192] mode=indexing
                  tunnel: w164 -> [w191] mode=indexing
                  tunnel: [w190] -> w163 mode=indexing
                  n111 = Bundle By Name(cluster=T6 {"Pin name"="", "Vertical range"=10.0, "Vertical offset"=0.0, "Probe attenuation"=1.0, "Vertical coupling"=1, "Channel enabled"=TRUE, "Input impedance"=0, "Max input frequency"=0.0, "Min sample rate"=20000000.0, "Reference position"=50.0, "Min record length"=1000, "Enforce realtime"=TRUE} ("Scope Parameters"), "Pin name"=w202, "Vertical range"=w201, "Vertical offset"=w200, "Probe attenuation"=w199, "Vertical coupling"=w198, "Channel enabled"=w197, "Input impedance"=w196, "Max input frequency"=w195, "Min sample rate"=w194, "Reference position"=w193, "Min record length"=w192, "Enforce realtime"=w191) -> (w190:T6)
                }
                n112 = call "Scope Settings Dialog.vi"("Scope Parameters"=w163) -> ("Scope Parameters out"=w188:T6[])  [unwired: 10 in]
                n113 = for {
                  tunnel: w188 -> [w215] mode=indexing
                  tunnel: [w214] -> w185 mode=indexing
                  tunnel: [w213] -> w187 mode=indexing
                  tunnel: [w212] -> w184 mode=indexing
                  tunnel: [w211] -> w183 mode=indexing
                  tunnel: [w210] -> w186 mode=indexing
                  tunnel: [w209] -> w182 mode=indexing
                  tunnel: [w208] -> w181 mode=indexing
                  tunnel: [w207] -> w180 mode=indexing
                  tunnel: [w206] -> w179 mode=indexing
                  tunnel: [w205] -> w178 mode=indexing
                  tunnel: [w204] -> w177 mode=indexing
                  tunnel: [w203] -> w176 mode=indexing
                  n114 = Unbundle By Name(w215) -> ("Pin name"=w214:string, "Vertical range"=w213:dbl, "Vertical offset"=w212:dbl, "Probe attenuation"=w211:dbl, "Vertical coupling"=w210:i32, "Channel enabled"=w209:bool, "Input impedance"=w208:u32, "Max input frequency"=w207:dbl, "Min sample rate"=w206:dbl, "Reference position"=w205:dbl, "Min record length"=w204:i32, "Enforce realtime"=w203:bool)
                }
                n115 = property on="Pin Names for Scope" class="Arr (strict)"("Value"=w185) -> ()  [unwired: 2 in, 2 out]
                n116 = property on="vertical range" class="Arr (strict)"("Value"=w187) -> ()  [unwired: 2 in, 2 out]
                n117 = property on="vertical offset" class="Arr (strict)"("Value"=w184) -> ()  [unwired: 2 in, 2 out]
                n118 = property on="probe attenuation" class="Arr (strict)"("Value"=w183) -> ()  [unwired: 2 in, 2 out]
                n119 = property on="vertical coupling" class="Arr (strict)"("Value"=w186) -> ()  [unwired: 2 in, 2 out]
                n120 = property on="channel enabled" class="Arr (strict)"("Value"=w182) -> ()  [unwired: 2 in, 2 out]
                n121 = property on="input impedance" class="Arr (strict)"("Value"=w181) -> ()  [unwired: 2 in, 2 out]
                n122 = property on="max input frequency" class="Arr (strict)"("Value"=w180) -> ()  [unwired: 2 in, 2 out]
                n123 = property on="min sample rate" class="Arr (strict)"("Value"=w179) -> ()  [unwired: 2 in, 2 out]
                n124 = property on="reference position" class="Arr (strict)"("Value"=w178) -> ()  [unwired: 2 in, 2 out]
                n125 = property on="min record length" class="Arr (strict)"("Value"=w177) -> ()  [unwired: 2 in, 2 out]
                n126 = property on="enforce realtime" class="Arr (strict)"("Value"=w176) -> ()  [unwired: 2 in, 2 out]
              }
              event "Open DMM Dialog": Value Change {
                n127 = event-data() -> ()  [unwired: 1 in, 6 out]
                n128 = property on="dmm pin names" class="Arr (strict)"() -> ("Value"=w224:string[])  [unwired: 2 in, 2 out]
                n129 = property on="dmm function array" class="Arr (strict)"() -> ("Value"=w223:u32[])  [unwired: 2 in, 2 out]
                n130 = property on="dmm resolution in digits array" class="Arr (strict)"() -> ("Value"=w222:T3[])  [unwired: 2 in, 2 out]
                n131 = property on="dmm range array" class="Arr (strict)"() -> ("Value"=w221:dbl[])  [unwired: 2 in, 2 out]
                n132 = for {
                  tunnel: [w235] -> w225 mode=indexing
                  tunnel: w224 -> [w234] mode=indexing
                  tunnel: w223 -> [w233] mode=indexing
                  tunnel: w222 -> [w232] mode=indexing
                  tunnel: w221 -> [w231] mode=indexing
                  n133 = Bundle By Name(cluster=T7 {"Pin name"="", "Function"=0, "Resolution in Digits"=5.5, "Range"=10.0} ("Scope Parameters"), "Pin name"=w234, "Function"=w233, "Resolution in Digits"=w232, "Range"=w231) -> (w235:T7)
                }
                n134 = call "DMM Settings Dialog.vi"("DMM Parameters"=w225) -> ("DMM Parameters out"=w220:T7[])  [unwired: 10 in]
                n135 = for {
                  tunnel: w220 -> [w230] mode=indexing
                  tunnel: [w229] -> w218 mode=indexing
                  tunnel: [w228] -> w219 mode=indexing
                  tunnel: [w227] -> w217 mode=indexing
                  tunnel: [w226] -> w216 mode=indexing
                  n136 = Unbundle By Name(w230) -> ("Pin name"=w229:string, "Function"=w228:u32, "Resolution in Digits"=w227:dbl, "Range"=w226:dbl)
                }
                n137 = property on="dmm pin names" class="Arr (strict)"("Value"=w218) -> ()  [unwired: 2 in, 2 out]
                n138 = property on="dmm function array" class="Arr (strict)"("Value"=w219) -> ()  [unwired: 2 in, 2 out]
                n139 = property on="dmm resolution in digits array" class="Arr (strict)"("Value"=w217) -> ()  [unwired: 2 in, 2 out]
                n140 = property on="dmm range array" class="Arr (strict)"("Value"=w216) -> ()  [unwired: 2 in, 2 out]
              }
              event "Use Source voltage array": Value Change {
                n141 = event-data() -> ("NewVal"=w237:bool)  [unwired: 1 in, 5 out]
                n142 = case shown="True" w237 {
                  frame False {
                    w238 = T8."Enabled" ("Disabled")
                    n143 = property on="Source start voltage array" class="Arr (strict)"("DisabledEnum"=w238) -> ()  [unwired: 2 in, 2 out]
                    n144 = property on="Source stop voltage array" class="Arr (strict)"("DisabledEnum"=w238) -> ()  [unwired: 2 in, 2 out]
                    n145 = property on="Source voltage array" class="Arr (strict)"("DisabledEnum"=T8."Disabled and Grayed Out" ("Disabled")) -> ()  [unwired: 2 in, 2 out]
                    n146 = property on="Source voltage sweep points" class="DigNum (strict)"("DisabledEnum"=w238) -> ()  [unwired: 2 in, 2 out]
                  }
                  frame True {
                    w241 = T8."Disabled and Grayed Out" ("Disabled")
                    n147 = property on="Source start voltage array" class="Arr (strict)"("DisabledEnum"=w241) -> ()  [unwired: 2 in, 2 out]
                    n148 = property on="Source stop voltage array" class="Arr (strict)"("DisabledEnum"=w241) -> ()  [unwired: 2 in, 2 out]
                    n149 = property on="Source voltage array" class="Arr (strict)"("DisabledEnum"=T8."Enabled" ("Disabled")) -> ()  [unwired: 2 in, 2 out]
                    n150 = property on="Source voltage sweep points" class="DigNum (strict)"("DisabledEnum"=w241) -> ()  [unwired: 2 in, 2 out]
                  }
                }
              }
              event "Use Load current array": Value Change {
                n151 = event-data() -> ("NewVal"=w242:bool)  [unwired: 1 in, 5 out]
                n152 = case shown="True" w242 {
                  frame False {
                    w244 = T8."Enabled" ("Disabled")
                    n153 = property on="Load sweep type" class="CmbBox"("DisabledEnum"=w244) -> ()  [unwired: 2 in, 2 out]
                    n154 = property on="Load start current" class="DigNum (strict)"("DisabledEnum"=w244) -> ()  [unwired: 2 in, 2 out]
                    n155 = property on="Load stop current" class="DigNum (strict)"("DisabledEnum"=w244) -> ()  [unwired: 2 in, 2 out]
                    n156 = property on="Load current sweep points/points per decade" class="DigNum (strict)"("DisabledEnum"=w244) -> ()  [unwired: 2 in, 2 out]
                    n157 = property on="Load current array" class="Arr (strict)"("DisabledEnum"=T8."Disabled and Grayed Out" ("Disabled")) -> ()  [unwired: 2 in, 2 out]
                  }
                  frame True {
                    w246 = T8."Disabled and Grayed Out" ("Disabled")
                    n158 = property on="Load sweep type" class="CmbBox"("DisabledEnum"=w246) -> ()  [unwired: 2 in, 2 out]
                    n159 = property on="Load start current" class="DigNum (strict)"("DisabledEnum"=w246) -> ()  [unwired: 2 in, 2 out]
                    n160 = property on="Load stop current" class="DigNum (strict)"("DisabledEnum"=w246) -> ()  [unwired: 2 in, 2 out]
                    n161 = property on="Load current sweep points/points per decade" class="DigNum (strict)"("DisabledEnum"=w246) -> ()  [unwired: 2 in, 2 out]
                    n162 = property on="Load current array" class="Arr (strict)"("DisabledEnum"=T8."Enabled" ("Disabled")) -> ()  [unwired: 2 in, 2 out]
                  }
                }
              }
              event "Source voltage array": Value Change {
                n163 = event-data() -> ()  [unwired: 1 in, 6 out]
                n164 = property on="Source voltage array" class="Arr (strict)"() -> ("Value"=w250:dbl[][])  [unwired: 2 in, 2 out]
                n165 = Array Size(array=w250) -> (size(s)=w247:i32[])
                n166 = Multiply Array Elements(1:w247) -> (0:w249:i32)
                n167 = Reshape Array(w250, w249) -> (w248:dbl[])
                n168 = property on="Source voltage concatenated array" class="Arr (strict)"("Value"=w248) -> ()  [unwired: 2 in, 2 out]
                n169 = property on="Source voltage array size" class="Arr (strict)"("Value"=w247) -> ()  [unwired: 2 in, 2 out]
              }
              event Panel Close? {
                n170 = event-data() -> ()  [unwired: 1 in, 4 out]
                n171 = Enqueue Element(queue=w252, element="Exit", error in (no error)=w254) -> (error out=w253:errorcluster)  [unwired: 1 in, 2 out]
                n172 = event-data("Discard?"=TRUE) -> ()  [unwired: 1 in, 1 out]
              }
            }
          }
          frame "Initialize" {
            n173 = for {
              tunnel: w261 -> [w263] mode=indexing
              n174 = property class="XYGraph (strict)"(reference=w263, "ActPaletteTool"=2 ("Palette:Active Tool")) -> ()  [unwired: 1 in, 2 out]
            }
            n175 = property on="Status" class="Str"("Visible"=FALSE) -> (error out=w258:errorcluster)  [unwired: 2 in, 1 out]
            n176 = call "Stall Data Flow.vim"("value in"=w258, "milliseconds to wait"=u32 500) -> ("value out"=w257:errorcluster)  [unwired: 1 out]
            n177 = property on="Mode of operation" class="Enum (strict)"(error in=w257, "Val(Sgnl)"=T5."Power on the DUT" ("Value (Signaling)")) -> ()  [unwired: 1 in, 2 out]
          }
          frame "Post UI Update" {
            w281 = u32[] [15787074, 5682409, 15535092, 40563, 13983232, 35009, 15113984, 13400487, 15993633, 10221451, 8148942, 15869817, 32914, 10196480, 6271923, 16355671]  # Plot colors
            # "-Sets various properties of graphs like color, point style, plot name etc.\n-Increases the legend number of rows if the voltage values are less than 4 and \nif it is greater than 4 then make the default rows as 4 and enable the vertical scrollbar.\n-Also sets the plot minimum property to source sweep points which disables the unused plots in the graph."
            # "Plot the deleted array in the graph"
            # "This case will be triggered, after framework updates the User interface with result values."
            n178 = local read "Source sweep points"() -> (w280:i32)
            n179 = local read "Voltage values"() -> (w278:dbl[])
            n180 = for {
              tunnel: w278 -> [w321]
              tunnel: [w320] -> w279
              tunnel: w282 -> [w319] mode=indexing
              tunnel: w280 -> [w318]
              tunnel: w281 -> [w317]
              n181 = for {
                tunnel: w321 -> [w334] mode=indexing
                tunnel: [w334] -> w320 mode=indexing
                tunnel: w319 -> [w327]
                tunnel: w318 -> [w324]
                tunnel: w317 -> [w330] mode=indexing
                i -> [w328]
                n182 = Greater?(x=w328, y=3) -> (0:w332:bool)
                n183 = To Unsigned Long Integer(number=w328) -> (unsigned 32bit integer=w331:u32)
                n184 = Increment(x=w328) -> (x+1=w326:i32)
                n185 = Format Value(format string="%.3f", value (0)=w334) -> (output string=w337:string)  [unwired: 1 out]
                n186 = case shown="False" w332 {
                  tunnel: w327 -> [w343 w349]
                  tunnel: w326 -> [w342 _]
                  tunnel: [w341 w348] -> w325
                  tunnel: w324 -> [w339 w344]
                  tunnel: [w340 w347] -> w323
                  frame False {
                    n187 = property on="Property Node" class="XYGraph (strict)"(reference=w343, "LegScrollVis"=FALSE ("Legend:Scrollbar Visible"), "LegNumRows"=w342, "LegPlotMin"=w339) -> (reference out=w341:refnum<vi>, error out=w340:errorcluster)  [unwired: 1 in]
                  }
                  frame True {
                    n188 = property on="Property Node" class="XYGraph (strict)"(reference=w349, "LegScrollVis"=TRUE ("Legend:Scrollbar Visible"), "LegNumRows"=u32 4 ("Legend:Number of Rows"), "LegPlotMin"=w344) -> (reference out=w348:refnum<vi>, error out=w347:errorcluster)  [unwired: 1 in]
                  }
                }
                n189 = Concatenate Strings(" Vin = " ("string"), w337) -> (w322:string)
                n190 = property on="Property Node" class="XYGraph (strict)"(reference=w325, error in=w323, "Active Plot"=w331, "Plot.Point Style"=u8 5, "Plot.Plot Color"=w330, "Plot.Fill/Pt. Color"=w330, "Plot.Plot Name"=w322) -> ()  [unwired: 2 out]
              }
            }
            n191 = local read "Maximum load regulation"() -> (w273:dbl[])
            n192 = local read "Minimum load regulation"() -> (w274:dbl[])
            n193 = local read "Maximum load voltage"() -> (w275:dbl[])
            n194 = local read "Minimum load voltage"() -> (w276:dbl[])
            n195 = local read "Maximum efficiency"() -> (w277:dbl[])
            n196 = Array Size(array=w279) -> (size(s)=w289:i32)
            n197 = local read "Load voltage deviation"() -> (w291:dbl[])
            n198 = local read "Load sweep points"() -> (w286:i32)
            n199 = local read "Load voltages"() -> (w290:dbl[])
            n200 = local read "Load currents"() -> (w288:dbl[])
            n201 = local read "Efficiency"() -> (w287:dbl[])
            n202 = for {
              N: w289 -> [_]
              tunnel: [w366] -> w283 mode=indexing
              tunnel: [w365] -> w284 mode=indexing
              tunnel: [w364] -> w285 mode=indexing
              tunnel: w286 -> [w351]
              shift-right: [w359] -> _
              shift-left: w288 -> [w363]
              shift-right: [w357] -> _
              shift-left: w287 -> [w362]
              shift-right: [w356] -> _
              shift-left: w290 -> [w361]
              shift-right: [w355] -> _
              shift-left: w291 -> [w360]
              w350 = 0 ("index")
              n203 = Delete From Array(array=w363, length=w351, index=w350) -> (deleted portion=w358:dbl[], array with subset deleted=w359:dbl[])
              n204 = Delete From Array(array=w362, length=w351, index=w350) -> (deleted portion=w352:dbl[], array with subset deleted=w357:dbl[])
              n205 = Delete From Array(array=w361, length=w351, index=w350) -> (deleted portion=w353:dbl[], array with subset deleted=w356:dbl[])
              n206 = Delete From Array(array=w360, length=w351, index=w350) -> (deleted portion=w354:dbl[], array with subset deleted=w355:dbl[])
              n207 = Bundle("Load currents"=w358, "Efficiency"=w352) -> (w366:T10)  [unwired: 1 in]
              n208 = Bundle("Load currents"=w358, "Load voltages"=w353) -> (w365:T11)  [unwired: 1 in]
              n209 = Bundle("Load currents"=w358, "Load voltage deviation"=w354) -> (w364:T12)  [unwired: 1 in]
            }
            "EfficiencyGraph" <- w283
            "LoadRegulationGraph(V/A)" <- w284
            "LoadRegulationGraph(%)" <- w285
            n210 = for {
              tunnel: w276 -> [w314] mode=indexing
              tunnel: [w316] -> w272 mode=indexing
              tunnel: w277 -> [w315] mode=indexing
              tunnel: w275 -> [w313] mode=indexing
              tunnel: w274 -> [w312] mode=indexing
              tunnel: w278 -> [w308] mode=indexing
              tunnel: w273 -> [w303] mode=indexing
              w305 = "%0.9f" ("initial string")
              w304 = "| " ("initial string")
              n211 = Format Into String(format string=w305, w308) -> (resulting string=w307:string)  [unwired: 2 in, 1 out]
              n212 = Format Into String(format string=w305, initial string=w304, w315) -> (resulting string=w311:string)  [unwired: 1 in, 1 out]
              n213 = Format Into String(format string=w305, initial string=w304, w314) -> (resulting string=w310:string)  [unwired: 1 in, 1 out]
              n214 = Format Into String(format string=w305, initial string=w304, w313) -> (resulting string=w309:string)  [unwired: 1 in, 1 out]
              n215 = Format Into String(format string=w305, initial string=w304, w312) -> (resulting string=w306:string)  [unwired: 1 in, 1 out]
              n216 = Format Into String(format string=w305, initial string=w304, w303) -> (resulting string=w302:string)  [unwired: 1 in, 1 out]
              n217 = Build Array(w307, w311, w310, w309, w306, w302) -> (w316:string[])
            }
            "MeasTable" <- w272
            n218 = local read "concatenated waveform Y"() -> (w268:dbl[])
            n219 = local read "waveform length array"() -> (w270:i32[])
            n220 = local read "waveform t0 array"() -> (w271:dbl[])
            n221 = local read "waveform dt array"() -> (w269:dbl[])
            n222 = local read "waveform pins"() -> (w266:string[])
            n223 = local read "waveform sites"() -> (w265:i32[])
            n224 = for {
              N -> [w298]
              tunnel: w266 -> [w301] mode=indexing
              tunnel: w265 -> [w300] mode=indexing
              i -> [w295]
              n225 = Format Into String(format string="%s, Site %d", w301, w300) -> (resulting string=w294:string)  [unwired: 2 in, 1 out]
              n226 = To Unsigned Long Integer(number=w298) -> (unsigned 32bit integer=w297:u32)
              n227 = To Unsigned Long Integer(number=w295) -> (unsigned 32bit integer=w296:u32)
              n228 = property on="EfficiencyGraph 2" class="XYGraph (strict)"("LegNumRows"=w297, "Active Plot"=w296, "Plot.Point Style"=u8 0, "Plot.Plot Name"=w294) -> ()  [unwired: 2 in, 2 out]
            }
            n229 = call "Create XY Graph from Concatenated Waveform.vi"("waveform t0 array"=w271, "waveform dt array"=w269, "waveform length array"=w270, "concatenated waveform Y"=w268) -> ("XY Graph Array"=→"EfficiencyGraph 2":cluster{"time":dbl[], "waveform":dbl[]}[])  [unwired: 11 in]
          }
          frame "Exit" {
            # "This case is triggered to close the User Interface from framework"
            n230 = Build Array (concatenate)(w370, w369, w368) -> (w367:refnum<vi>[])
            n231 = Close Reference(reference=w367) -> (error out=w373:errorcluster)  [unwired: 1 in]
            n232 = Flush Queue(queue=w377, error in (no error)=w379) -> (queue out=w376:refnum<queue>, error out=w375:errorcluster)  [unwired: 1 out]
            n233 = Release Queue(queue=w376, force destroy? (F)=TRUE, error in (no error)=w375) -> (error out=w372:errorcluster)  [unwired: 2 out]
            n234 = Merge Errors(w373, w372) -> (w371:errorcluster)
          }
          frame "Handle Error" {
          }
        }
      }
    }
  }
